vi "Write Motion Controller .vi"(8 "error in (no error)":errorcluster, 10 "Motion Controller":refnum<class "iMotion Controller.lvclass">[](array[class]), 11 "MAS in":refnum<class "MAS.lvclass">) -> (0 "error out":errorcluster, 3 "MAS out":refnum<class "MAS.lvclass">)   [LabVIEW 2022 SP3, in "MAS.lvclass"]
uses:
  MAS.lvclass
  iMotion Controller/iMotion Controller.lvclass
  MAS.lvclass/MAS.ctl
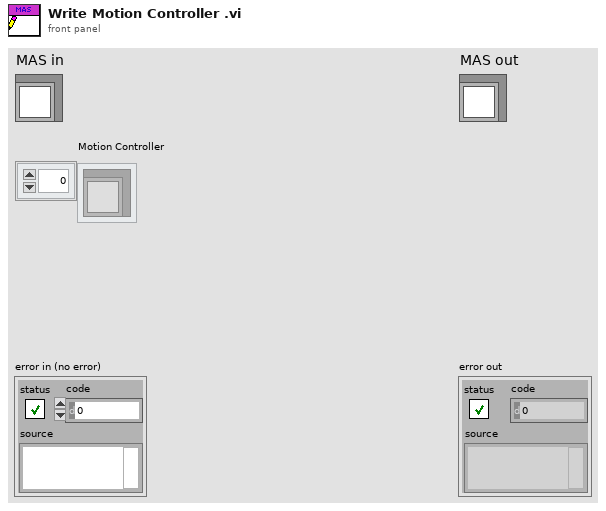
[diagram p1: front panel]
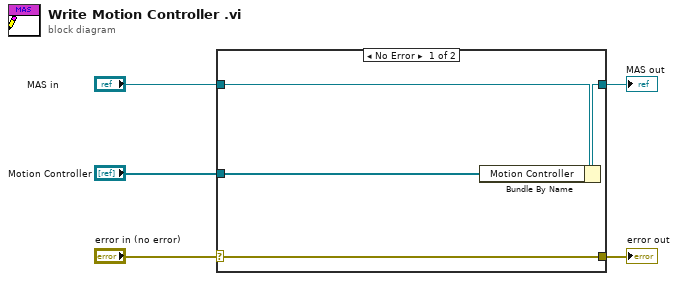
[diagram p0: block diagram]
diagram:
  n1 = case shown="No Error" "error in (no error)" {
    selector: "error in (no error)" -> [w9 w10]
    tunnel: [w9 w10] -> w4
    tunnel: [w7 w11] -> w2
    tunnel: "MAS in" -> [w8 w11]
    tunnel: "Motion Controller" -> [w6 _]
    frame No Error {
      n2 = Bundle By Name(cluster=w8, "Motion Controller"=w6) -> (w7:refnum<class "MAS.lvclass">)
    }
    frame Error {
    }
  }
  "error out" <- w4
  "MAS out" <- w2
